vi "parse_uint8_roslv.vi"   [LabVIEW 2014]
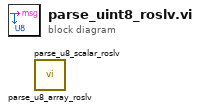
[diagram p0: block diagram]
diagram:
  n1 = call "parse_u8_array_roslv.vi"() -> ()  [unwired: 5 in, 3 out]
  n2 = call "parse_u8_scalar_roslv.vi"() -> ()  [unwired: 5 in, 3 out]
